vi "Flatten UIP Value.vi"(11 "UIP In":refnum<class "SizeUIP.lvclass">) -> (0 "Error Out":errorcluster, 2 "String Value":string, 3 "UIP Out":refnum<class "SizeUIP.lvclass">)   [LabVIEW 2015, in "SizeUIP.lvclass"]
uses:
  SizeUIP.lvclass
  SizeUIP.lvclass/SizeUIP.ctl
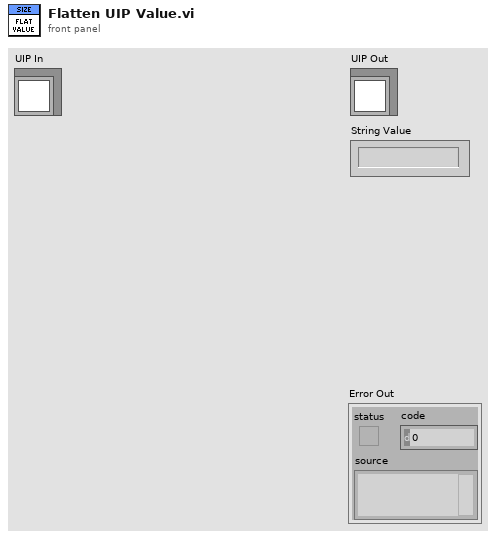
[diagram p1: front panel]
types:
  T1 = typedef "LVBoundsTypeDef.ctl" = cluster{"Width":u32, "Height":u32}
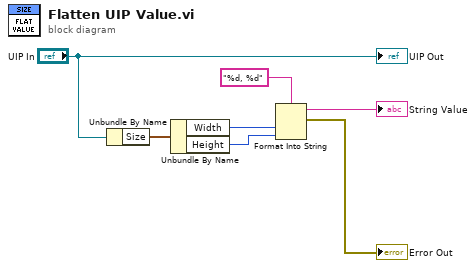
[diagram p0: block diagram]
diagram:
  n1 = Unbundle By Name("UIP In") -> ("Size"=w6:T1)
  n2 = Unbundle By Name(w6) -> ("Width"=w5:u32, "Height"=w4:u32)
  n3 = Format Into String(format string="%d, %d", w5, w4) -> (resulting string=→"String Value":string, error out=→"Error Out":errorcluster)  [unwired: 2 in]
  "UIP Out" <- "UIP In"
